vi "Menu Button Move Buttons and Reposition.vi"(8 "error in (no error)":errorcluster, 9 "Distance":i32) -> (0 "error out":errorcluster, 2 "Distance Moved":i32, 3 "User Interface References Out":T5)   [LabVIEW 2011]
uses:
  Framework SubVIs/Plugin Handler/Plugin Strict Type Definitions/Plugin Action Engine Enumerator Type Definition.ctl
  Parent Plugin Definition/Plugin Template/Generic Plugin.lvclass
  Menu Button Library/Menu Button xControl/Menu Button xControl.xctl
  Sliding Menu Type Definitions/User Interface Type Definitions.ctl
  <vilib>/Utility/config.llb/Config Data RefNum.ctl
  <vilib>/Utility/config.llb/NI_LVConfig.lvlib
  Button XControl.xctl
  Sliding Menu xControl/Sliding Menu State.ctl
  Sliding Menu xControl/Sliding Menu XControl.xctl
  Sliding Menu Type Definitions/Current User Action.ctl
  Sliding Menu Library.lvlib
  Sliding Menu xControl/Sliding Menu Methods.ctl
  Sliding Menu xControl/Sliding Menu Data.ctl
panel:
  in  "Display State In":T1
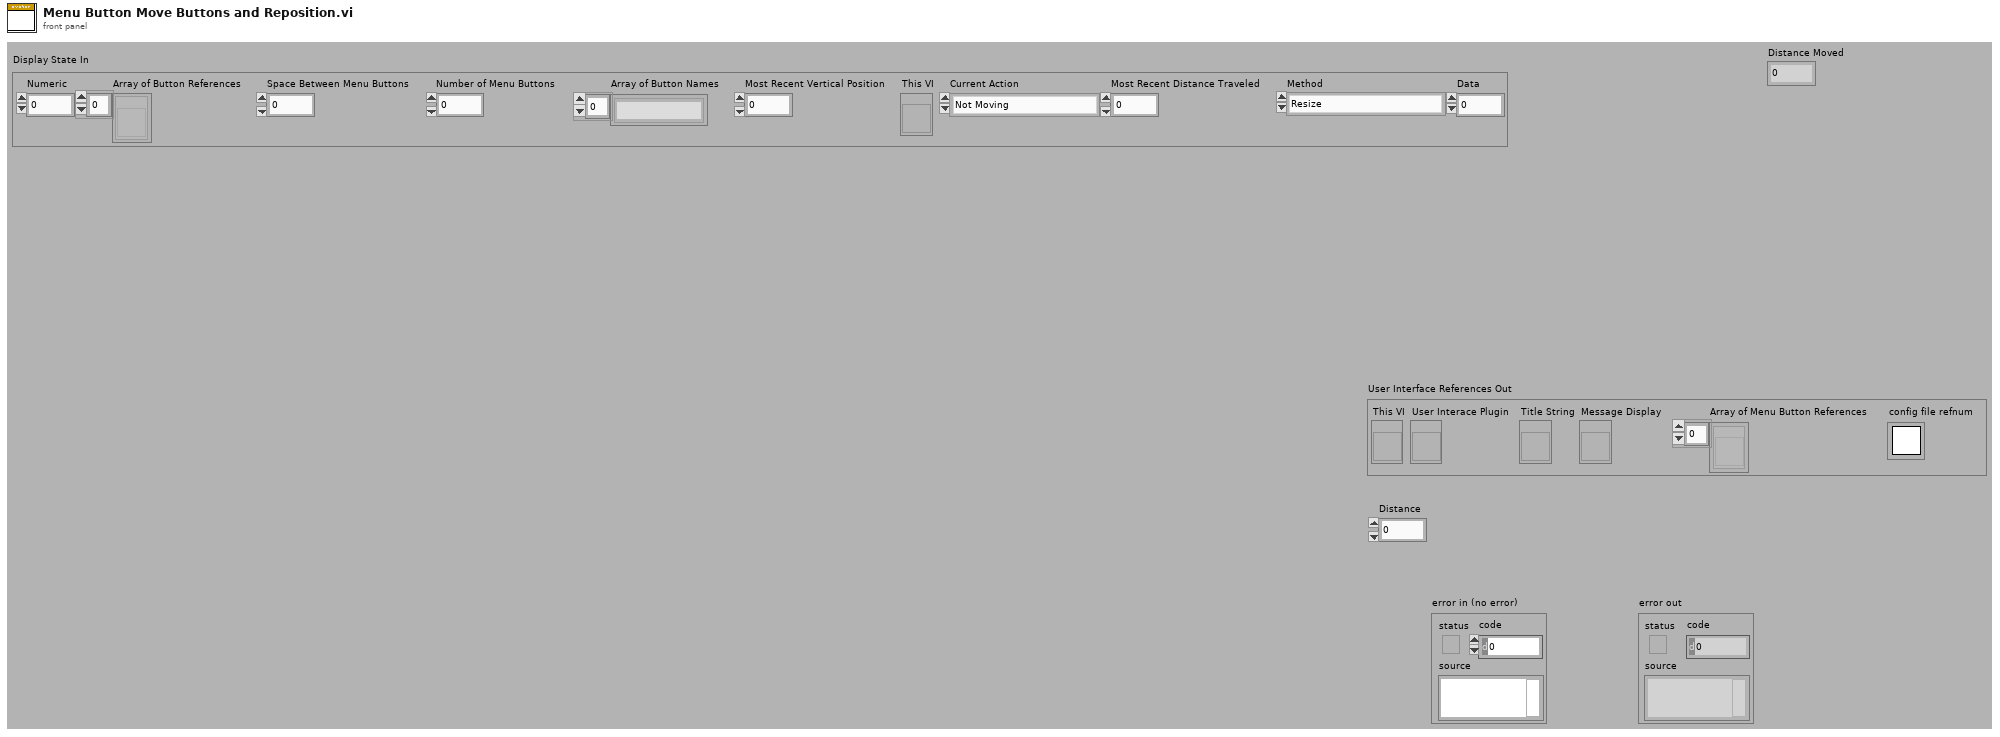
[diagram p1: front panel]
types:
  T1 = typedef "Sliding Menu Library.lvlib/Sliding Menu XControl.xctl/Sliding Menu State.ctl" = cluster{"Numeric":dbl, "Array of Button References":refnum<vi>[], "Space Between Menu Buttons":i32, "Number of Menu Buttons":i32, "Array of Button Names":string[], "Most Recent Vertical Position":i32, "This VI":refnum<vi>, "Current Action":T2, "Most Recent Distance Traveled":i32, "Method":T3, "Data In":T4}
  T2 = typedef "Sliding Menu Library.lvlib/Current User Action.ctl" = enum16{"Not Moving", "Mouse Down", "Mouse Up No Dragging", "Bounce Up Needed", "Bounce Down Needed", "Dragging", "Easing"}
  T3 = typedef "Sliding Menu Methods.ctl" = enum16{"Resize", "Move Up", "Move Down", "Move to 0"}
  T4 = typedef "Sliding Menu Library.lvlib/Sliding Menu XControl.xctl/Sliding Menu Data.ctl" = i32
  T5 = typedef "Sliding Menu Library.lvlib/User Interface Type Definitions.ctl" = cluster{"This VI":refnum<vi>, "User Interace Plugin":refnum<vi>, "Title String":refnum<vi>, "Message Display":refnum<vi>, "Array of Menu Button References":refnum<vi>[], "config file refnum":T6}
  T6 = typedef "NI_LVConfig.lvlib/Config Data RefNum.ctl" = refnum<k1>
  T7 = typedef "Plugin Action Engine Enumerator Type Definition.ctl" = enum16{"Initialize Test Data", "Get Entire Array", "Store Plugins"}
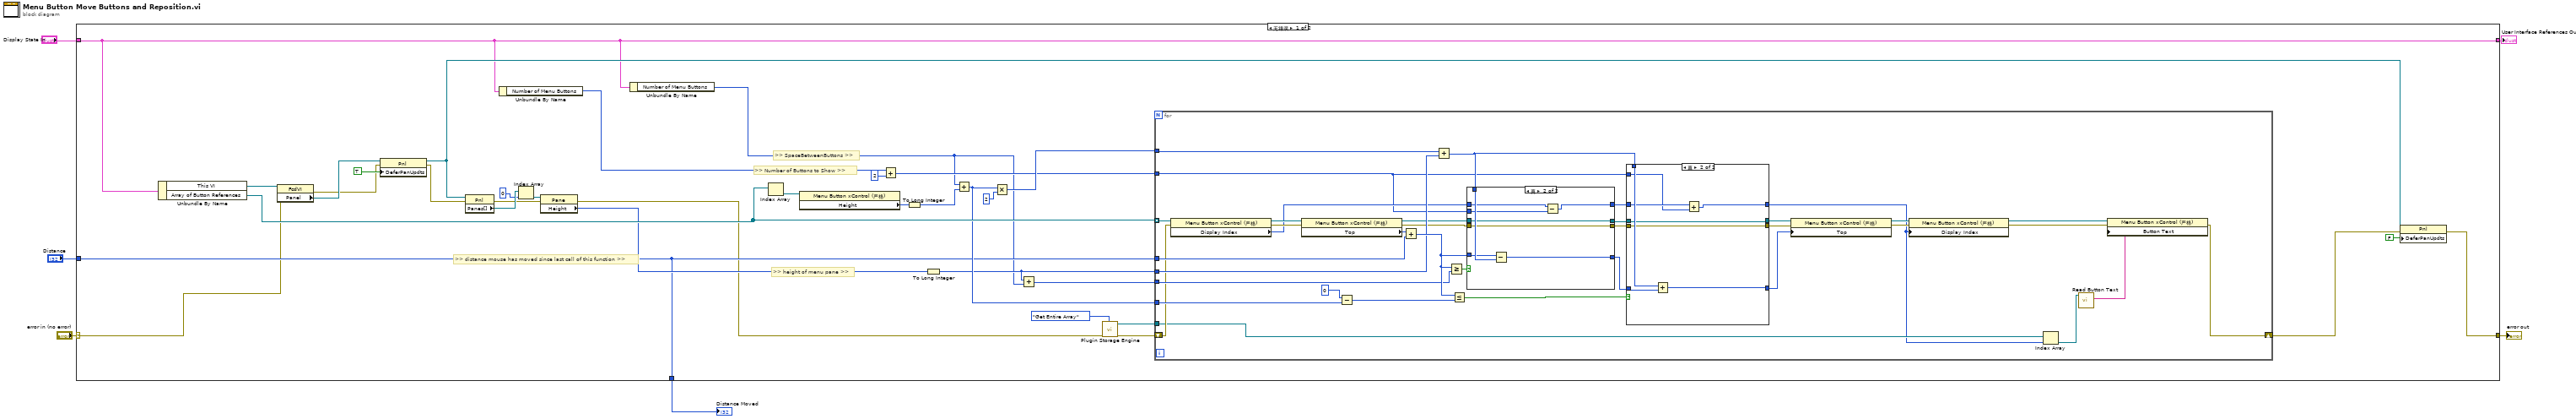
[diagram p0: block diagram]
diagram:
  n1 = case shown="无错误" "error in (no error)" {
    selector: "error in (no error)" -> [w12 w102]
    tunnel: [w7 w102] -> w6
    tunnel: [w11 w101] -> w4
    tunnel: "Display State In" -> [w11 w101]
    tunnel: "Distance" -> [w13 _]
    tunnel: [w13 _] -> w2
    frame No Error {
      # ">> Number of Buttons to Show >>"
      # ">> distance mouse has moved since last call of this function >>"
      # ">> height of menu pane >>"
      # ">> SpaceBetweenButtons >>"
      n2 = Unbundle By Name(w11) -> ("This VI"=w37:refnum<vi>, "Array of Button References"=w36:refnum<vi>[])
      n3 = property class="FcdVI"(reference=w37, error in=w12) -> (error out=w18:errorcluster, "Panel"=w20:refnum<vi>)  [unwired: 1 out]
      n4 = property class="Pnl"(reference=w20, error in=w18, "DeferPanUpdts"=TRUE ("Defer Panel Updates")) -> (reference out=w14:refnum<vi>, error out=w17:errorcluster)
      n5 = property class="Pnl"(reference=w14, error in=w17) -> (error out=w38:errorcluster, "Panes[]"=w40:refnum<vi>[])  [unwired: 1 out]
      n6 = Unbundle By Name(w11) -> ("Number of Menu Buttons"=w9:i32)
      n7 = Index Array(array=w40, index=0) -> (element=w21:refnum<vi>)
      n8 = property class="Pane"(reference=w21, error in=w38) -> (error out=w10:errorcluster, "Height"=w28:u32)  [unwired: 1 out]
      n9 = Unbundle By Name(w11) -> ("Number of Menu Buttons"=w8:i32)
      n10 = Index Array(array=w36) -> (element=w35:refnum<vi>)  [unwired: 1 in]
      n11 = property class="Menu Button xControl (严格)"(reference=w35) -> ("Height"=w34:u32)  [unwired: 1 in, 2 out]
      n12 = Add(x=w9, y=2) -> (x+y=w22:i32)
      n13 = To Long Integer(number=w34) -> (32bit integer=w32:i32)
      n14 = To Long Integer(number=w28) -> (32bit integer=w27:i32)
      n15 = Add(x=w8, y=w32) -> (x+y=w29:i32)
      n16 = Multiply(x=w29, y=2) -> (x*y=w30:i32)
      n17 = Add(x=w27, y=w8) -> (x+y=w26:i32)
      n18 = call "Plugin Storage Engine.vi"("Actions"=Plugin_Action_Engine_Enumerator_Type_Definition."Get Entire Array", "error in (no error)"=w10) -> ("error out"=w25:errorcluster, "Array of Plugins Out"=w23:refnum<class "Generic Plugin.lvclass">[])  [unwired: 8 in]
      n19 = for {
        tunnel: w36 -> [w56] mode=indexing
        tunnel: w13 -> [w75]
        shift-right: [w45] -> w15
        shift-left: w25 -> [w53]
        tunnel: w27 -> [w64]
        tunnel: w29 -> [w67]
        tunnel: w30 -> [w66]
        tunnel: w26 -> [w63]
        tunnel: w23 -> [w44]
        tunnel: w22 -> [w48]
        n20 = property class="Menu Button xControl (严格)"(reference=w56, error in=w53) -> (reference out=w55:refnum<vi>, error out=w54:errorcluster, "Display Index"=w50:i32)
        n21 = property class="Menu Button xControl (严格)"(reference=w55, error in=w54) -> (reference out=w62:refnum<vi>, error out=w61:errorcluster, "Top"=w76:i32)
        n22 = Subtract(x=0 ("y"), y=w67) -> (x-y=w68:i32)
        n23 = Add(x=w76, y=w75) -> (x+y=w74:i32)
        n24 = Add(x=w66, y=w64) -> (x+y=w65:i32)
        n25 = Greater Or Equal?(x=w74, y=w63) -> (x >= y?=w70:bool)
        n26 = Less Or Equal?(x=w74, y=w68) -> (x <= y?=w71:bool)
        n27 = case shown="真" w70 {
          tunnel: w74 -> [w92 w99]
          tunnel: [w92 w98] -> w72
          tunnel: w65 -> [_ w100]
          tunnel: w62 -> [w91 w97]
          tunnel: w61 -> [w90 w96]
          tunnel: [w91 w97] -> w60
          tunnel: [w90 w96] -> w59
          tunnel: w50 -> [w89 w95]
          tunnel: [w89 w94] -> w49
          tunnel: w48 -> [_ w93]
          frame False {
          }
          frame True {
            n28 = Subtract(x=w99, y=w100) -> (x-y=w98:i32)
            n29 = Subtract(x=w95, y=w93) -> (x-y=w94:i32)
          }
        }
        n30 = case shown="真" w71 {
          tunnel: [w80 w88] -> w73
          tunnel: w72 -> [w80 w86]
          tunnel: w65 -> [_ w87]
          tunnel: w60 -> [w79 w85]
          tunnel: w59 -> [w78 w84]
          tunnel: [w78 w84] -> w58
          tunnel: [w79 w85] -> w57
          tunnel: w49 -> [w77 w83]
          tunnel: [w77 w81] -> w43
          tunnel: w48 -> [_ w82]
          frame False {
          }
          frame True {
            n31 = Add(x=w87, y=w86) -> (x+y=w88:i32)
            n32 = Add(x=w83, y=w82) -> (x+y=w81:i32)
          }
        }
        n33 = property class="Menu Button xControl (严格)"(reference=w57, error in=w58, "Top"=w73) -> (reference out=w52:refnum<vi>, error out=w51:errorcluster)
        n34 = property class="Menu Button xControl (严格)"(reference=w52, error in=w51, "Display Index"=w43) -> (reference out=w47:refnum<vi>, error out=w46:errorcluster)
        n35 = Index Array(array=w44, index=w43) -> (element=w42:refnum<class "Generic Plugin.lvclass">)
        n36 = call-dynamic "Read Button Text.vi"("Generic Plugin in"=w42) -> ("Button Text"=w41:string)  [unwired: 8 in, 2 out]
        n37 = property class="Menu Button xControl (严格)"(reference=w47, error in=w46, "Button Text"=w41) -> (error out=w45:errorcluster)  [unwired: 1 out]
      }
      n38 = property class="Pnl"(reference=w14, error in=w15, "DeferPanUpdts"=FALSE ("Defer Panel Updates")) -> (error out=w7:errorcluster)  [unwired: 1 out]
    }
    frame Error {
    }
  }
  "error out" <- w6
  "User Interface References Out" <- w4
  "Distance Moved" <- w2
